vi "MAIN_SERVER.vi"() -> ()   [LabVIEW 2016]
uses:
  TypeDef/IN_Cluster.ctl
  TypeDef/OUT_CLUSTER.ctl
  <vilib>/DAQmx/read.llb/DAQmx Read (Analog 1D Wfm NChan NSamp).vi
  <vilib>/Analysis/baseanly.llb/Mean (DBL).vi
  <vilib>/DAQmx/miscellaneous.llb/DAQmx Fill In Error Info.vi
  <vilib>/Analysis/NI_AALBase.lvlib
  <vilib>/DAQmx/write.llb/DAQmx Write (Analog 1D DBL NChan 1Samp).vi
  <vilib>/DAQmx/read.llb/DAQmx Read (Analog 1D DBL NChan 1Samp).vi
  <vilib>/DAQmx/write.llb/DAQmx Write (Digital 1D Bool NChan 1Samp 1Line).vi
  <vilib>/DAQmx/read.llb/DAQmx Read (Digital 1D Bool NChan 1Samp 1Line).vi
panel:
  in  "Tab Control":enum32{"settings", "filtri AI ", "clusters"}(tab)
  in  "number of samples per channel":i32=500
  in  "rate":dbl=1000.0 format="%0.2f"
  out "Array nomi moduli":string[](array[string])
  in  "sample mode":i32(ring)=10123 items=["Finite Samples"=10178, "Continuous Samples"=10123, "Hardware Timed Single Point"=12522]
  in  "Impostazioni filtri digitali su AI":T1(array[cluster])=[{"filter?"=FALSE, "low cutoff freq: fl"=0.12500000000000006, "order"=2}, {"filter?"=FALSE, "low cutoff freq: fl"=0.12500000000000006, "order"=2}, {"filter?"=FALSE, "low cutoff freq: fl"=0.12500000000000006, "order"=2}, {"filter?"=FALSE, "low cutoff freq: fl"=0.12500000000000006, "order"=2}, {"filter?"=FALSE, "low cutoff freq: fl"=0.12500000000000006, "order"=2}, {"filter?"=FALSE, "low cutoff freq: fl"=0.12500000000000006, "order"=2}, {"filter?"=FALSE, "low cutoff freq: fl"=0.12500000000000006, "order"=2}, {"filter?"=FALSE, "low cutoff freq: fl"=0.12500000000000006, "order"=2}, {"filter?"=FALSE, "low cutoff freq: fl"=0.12500000000000006, "order"=2}, {"filter?"=FALSE, "low cutoff freq: fl"=0.12500000000000006, "order"=2}, {"filter?"=FALSE, "low cutoff freq: fl"=0.12500000000000006, "order"=2}, {"filter?"=FALSE, "low cutoff freq: fl"=0.12500000000000006, "order"=2}, {"filter?"=FALSE, "low cutoff freq: fl"=0.12500000000000006, "order"=2}, {"filter?"=FALSE, "low cutoff freq: fl"=0.12500000000000006, "order"=2}, {"filter?"=FALSE, "low cutoff freq: fl"=0.12500000000000006, "order"=2}, {"filter?"=FALSE, "low cutoff freq: fl"=0.12500000000000006, "order"=2}] {"low cutoff freq: fl" format="%0.4f"}
  out "AI Non filtrati":waveform(dbl)[](graph)
  out "AI filtrati":waveform(dbl)[](graph)
  out "Scritture":T2 {"AO" format="%f%0.2f"}
  in  "IN CLUSTER":T3 {"Stato uscite"."AO" format="%f%0.2f"; "AI2" format="%#_6f"; "TC" format="%#_4f"; "AI1" format="%#_6f"}
  in  "DO":bool[](array[boolean])
  in  "AO":dbl[](array[numeric]) format="%f%0.2f"
  in  "stop":bool
  # "AI"
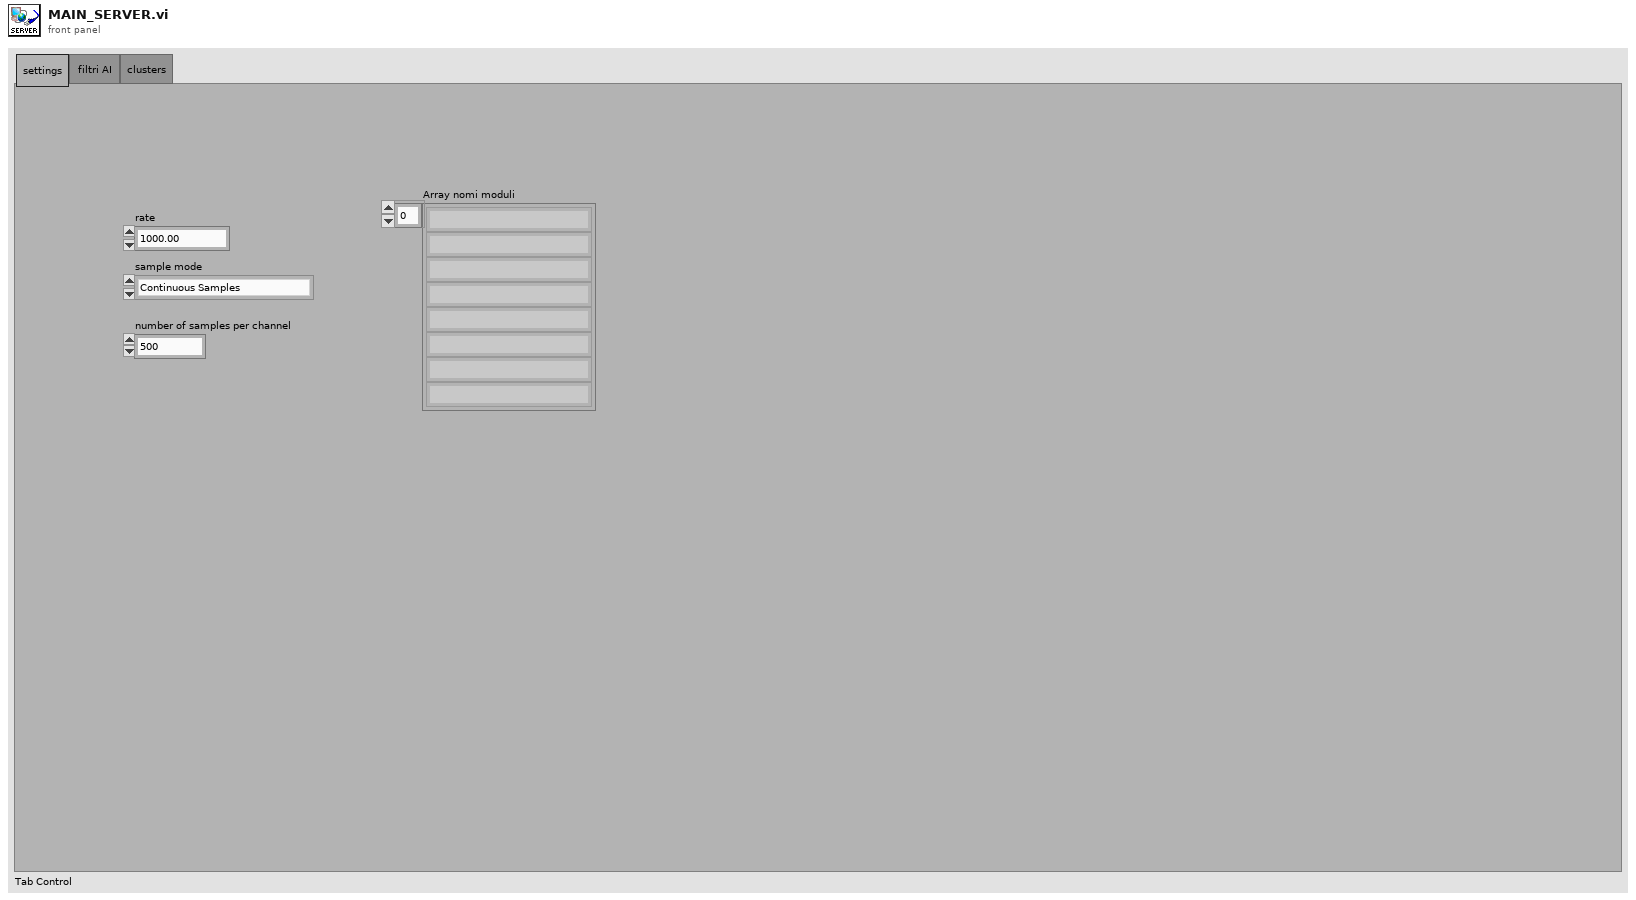
[diagram p1: front panel]
types:
  T1 = cluster{"filter?":bool, "low cutoff freq: fl":dbl, "order":i32}[]
  T2 = typedef "OUT_CLUSTER.ctl" = cluster{"DO ":bool[], "AO":dbl[], "Scelta banco PC1":dbl, "Scelta banco PC2":dbl, "Scelta ASP PC1":dbl, "Scelta ASP PC2":dbl, "Scelta MAND PC1":dbl, "Scelta MAND PC2":dbl, "Scelta Q PC1":dbl, "Scelta Q PC2":dbl}
  T3 = typedef "IN_Cluster.ctl" = cluster{"DI":bool[], "AI1":dbl[], "TC":dbl[], "AI2":dbl[], "Stato uscite":T2}
  T4 = cluster{"DI task":refnum<k21>, "DO task":refnum<k21>, "AI task":refnum<k21>, "AO task":refnum<k21>, "TC task":refnum<k21>}
  T5 = cluster{"Array of elements":cluster{"String":string, "variant":variant}[], "Single element":cluster{"String":string, "variant":variant}, "enque at\nopposite end (F)":bool, "no replications (F)":bool}
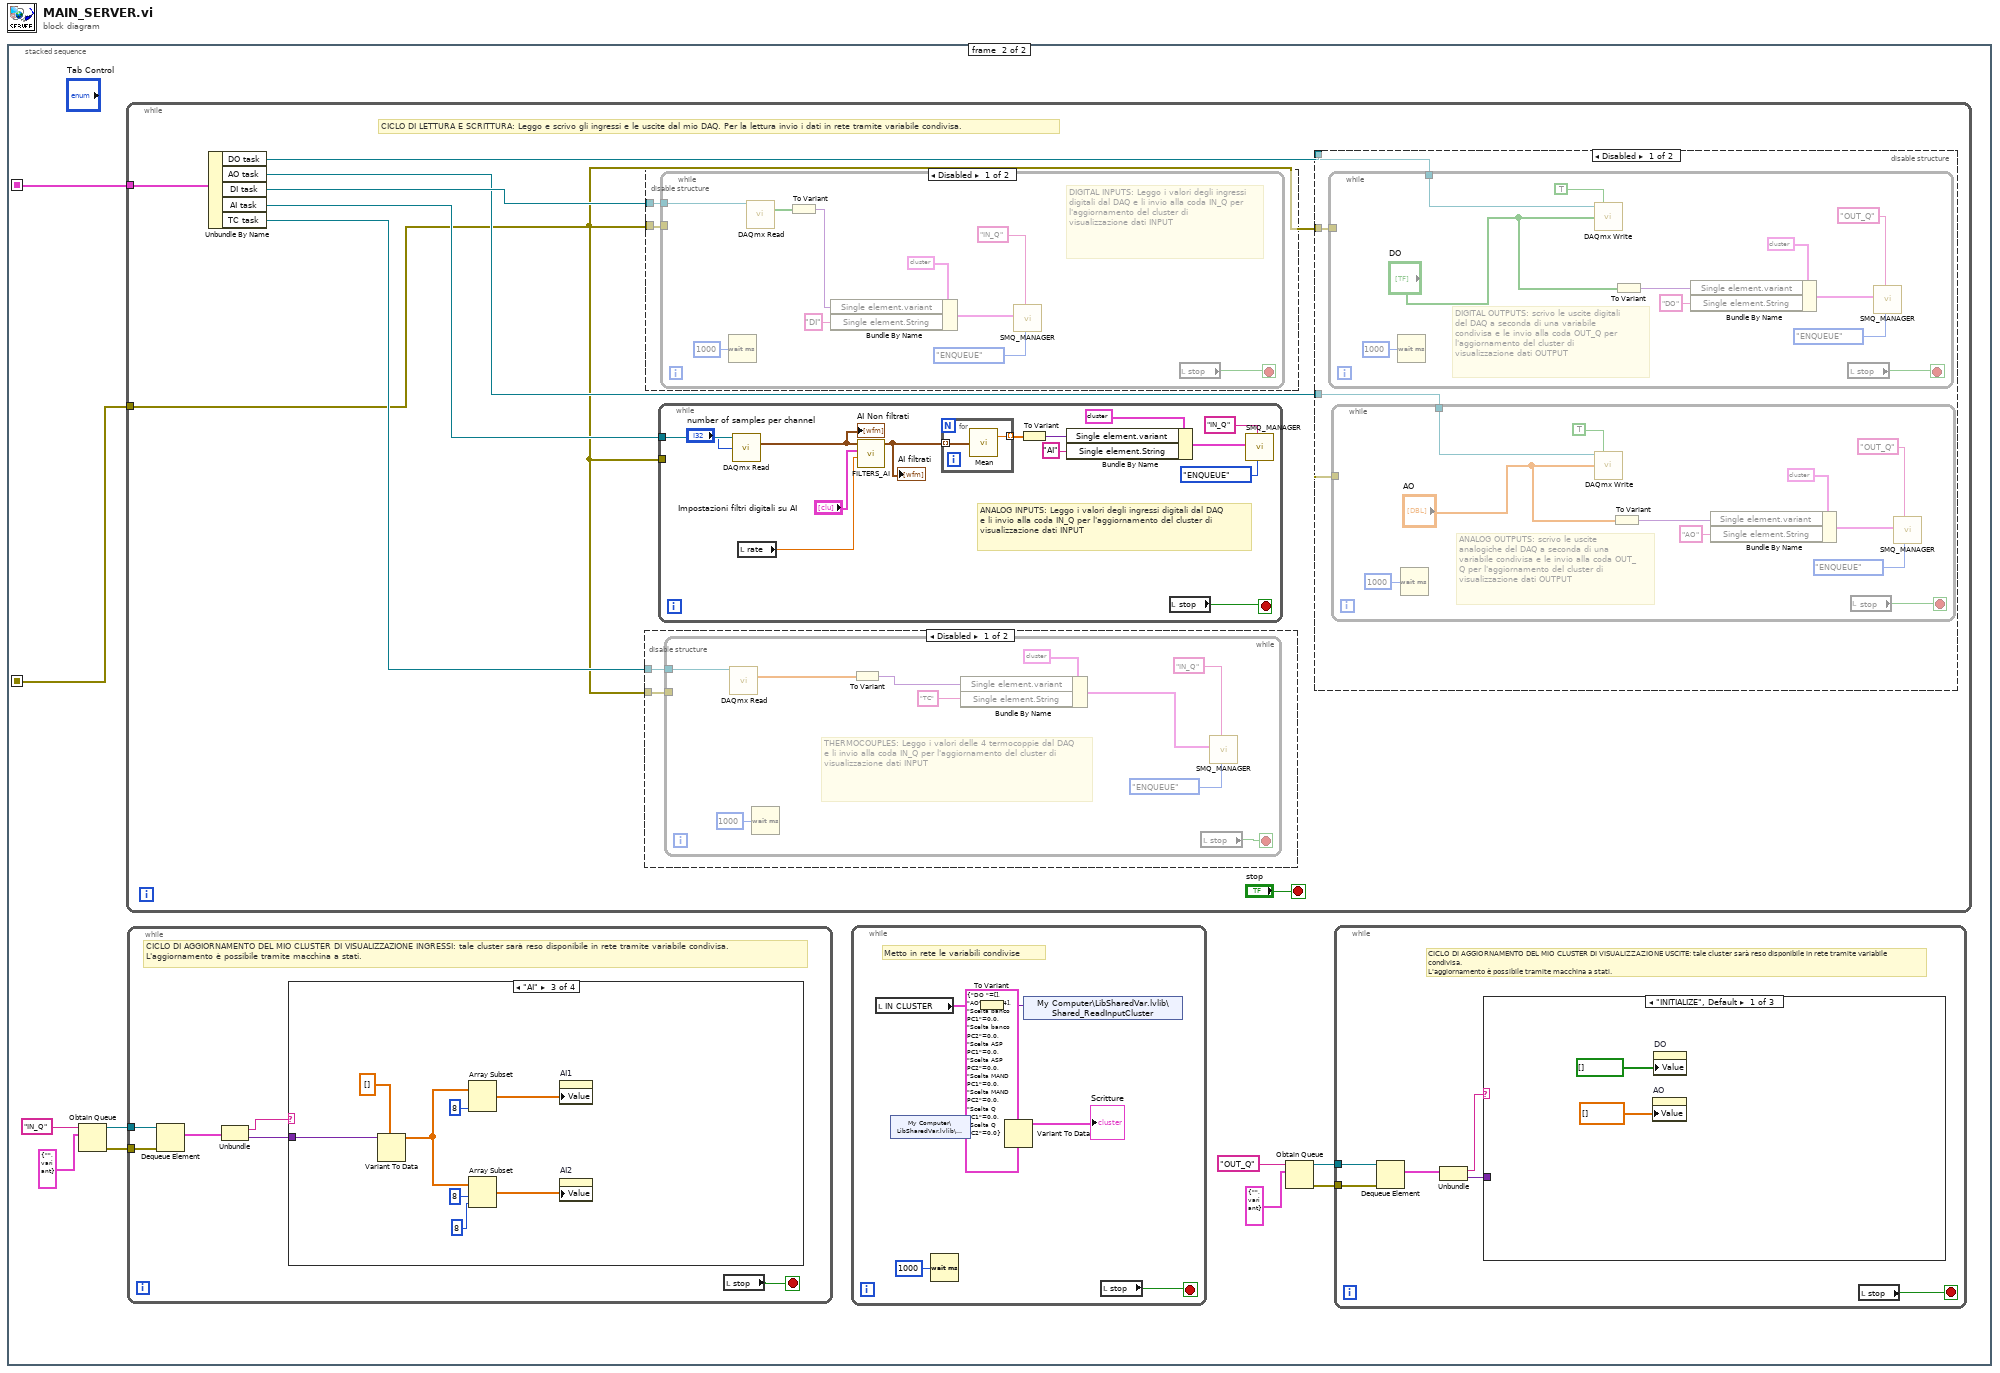
[diagram p0: block diagram]
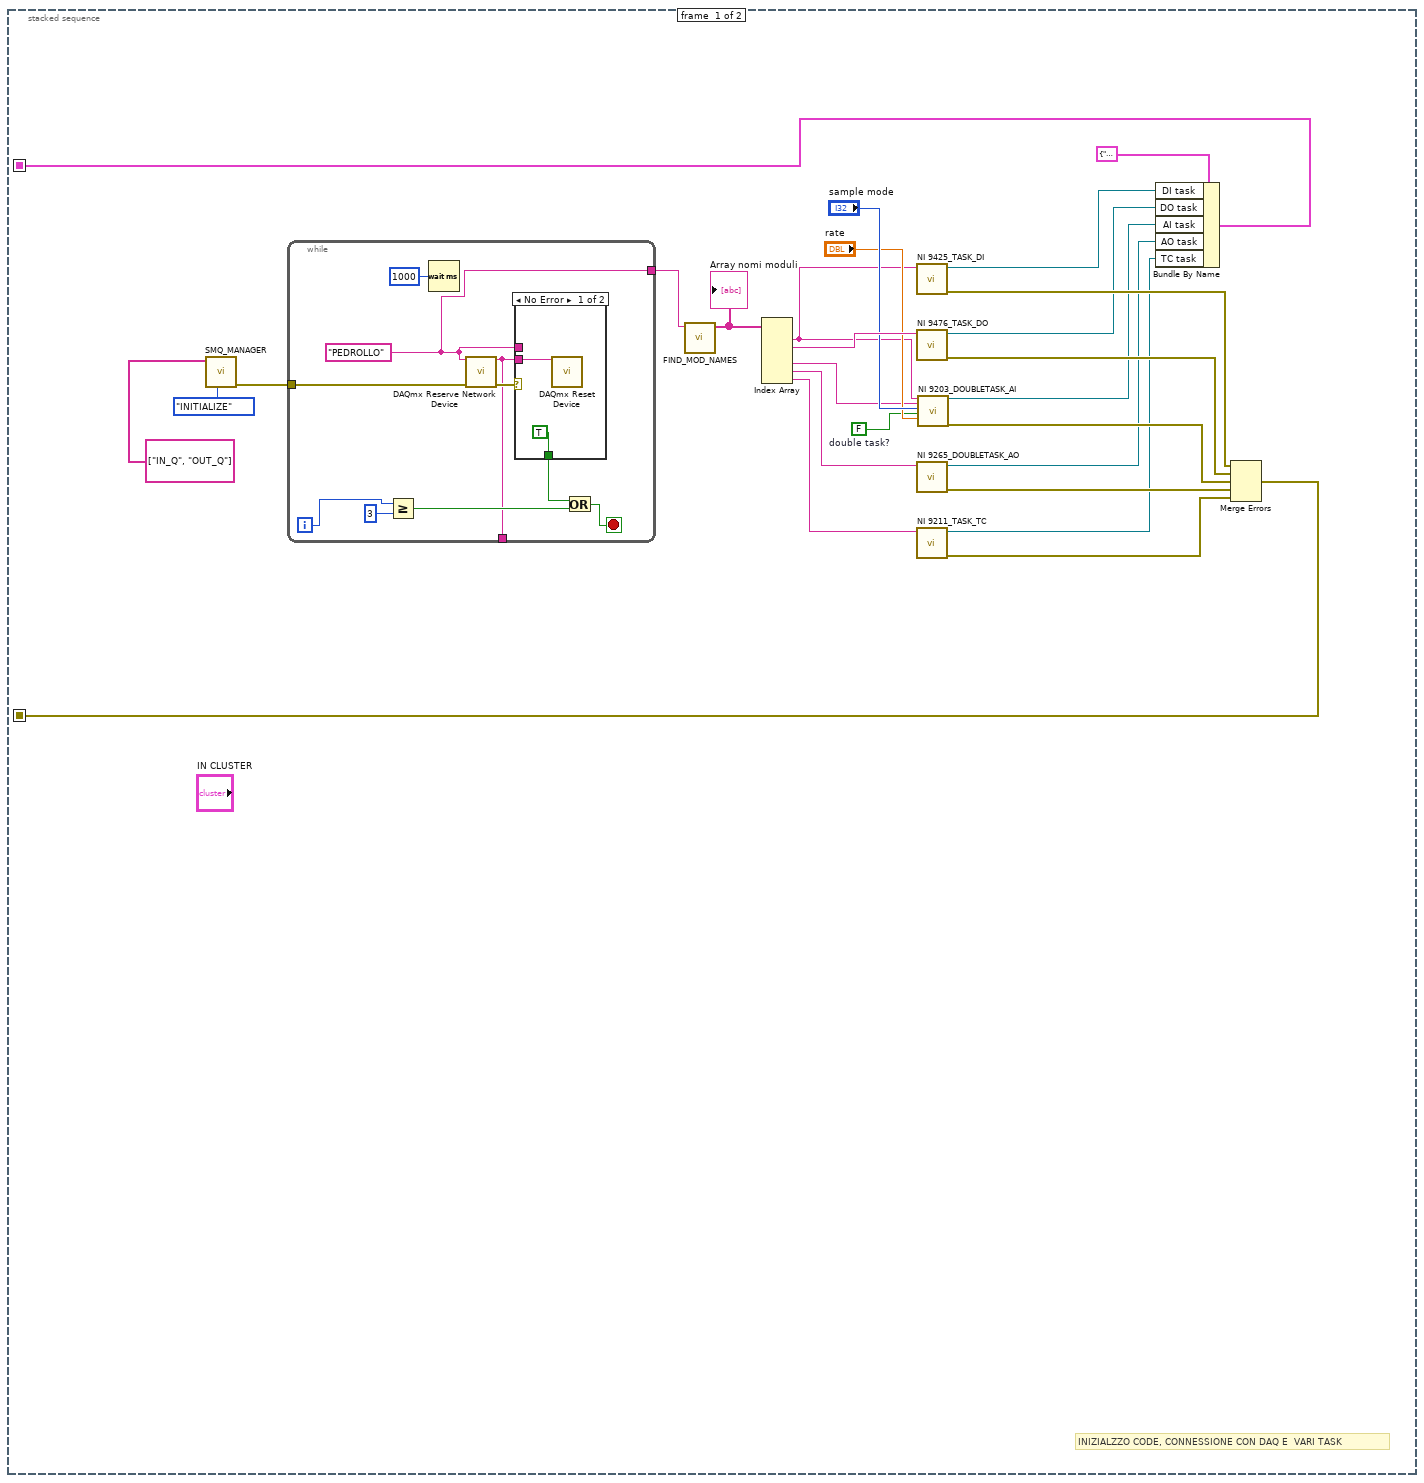
[diagram p2: hidden frame]
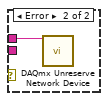
[diagram p3: hidden frame]
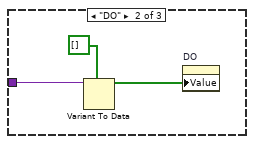
[diagram p4: hidden frame]
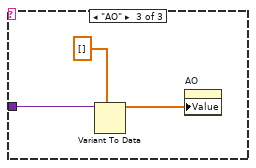
[diagram p5: hidden frame]
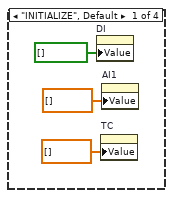
[diagram p6: hidden frame]
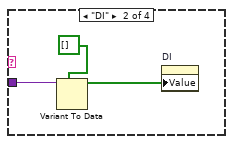
[diagram p7: hidden frame]
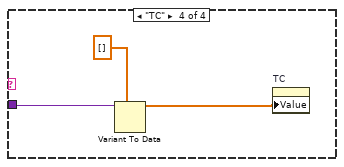
[diagram p8: hidden frame]
diagram:
  n1 = stacked-sequence {
    seq-local: [w16 _] -> [_ w49]
    seq-local: [w12 _] -> [_ w48]
    frame #0 {
      w2 = FALSE  # double task?
      # "INIZIALZZO CODE, CONNESSIONE CON DAQ E  VARI TASK"
      n2 = call <userlib>:"SMQ_MANAGER.vi"("Function"=enum16{"INITIALIZE", "ENQUEUE", "STOP ALL"}."INITIALIZE", "Queue array"=string[] ["IN_Q", "OUT_Q"]) -> ("error out"=w11:errorcluster)  [unwired: 9 in]
      n3 = while {
        tunnel: [w29] -> _
        tunnel: [w28] -> w17
        tunnel: w11 -> [w27]
        i -> [w34]
        stop <- w31 stop-if-true
        w28 = "PEDROLLO" ("RICERCA cDAQ")
        n4 = Greater Or Equal?(x=w34, y=3) -> (x >= y?=w32:bool)
        n5 = Wait (ms)(milliseconds to wait=u32 1000) -> ()  [unwired: 1 out]
        n6 = call <vilib>:"DAQmx Reserve Network Device.vi"("device in"=w28, "error in"=w27) -> ("device out"=w29:tag, "error out"=w36:errorcluster)  [unwired: 12 in]
        n7 = case shown="No Error" w36 {
          tunnel: w28 -> [_ w39]
          tunnel: [TRUE _] -> w35
          tunnel: w29 -> [w37 _]
          frame No Error {
            n8 = call <vilib>:"DAQmx Reset Device.vi"("device in"=w37) -> ()  [unwired: 14 in, 1 out]
          }
          frame Error {
            n9 = call <vilib>:"DAQmx Unreserve Network Device.vi"("device in"=w39) -> ()  [unwired: 13 in, 2 out]
          }
        }
        n10 = Or(x=w35, y=w32) -> (x .or. y?=w31:bool)
      }
      n11 = call "FIND_MOD_NAMES.vi"("RICERCA cDAQ"=w17) -> ("Array nomi moduli"=w23:string[])  [unwired: 7 in, 3 out]
      "Array nomi moduli" <- w23
      n12 = Index Array(array=w23) -> (element #1=w1:string, element #2=w24:string, element #4=w4:string, element #5=w6:string, element #6=w5:string)  [unwired: 6 in, 1 out]
      n13 = call "NI 9425_TASK_DI.vi"("MODULE NAME"=w1) -> ("error out"=w22:errorcluster, "task out"=w14:refnum<k21>)  [unwired: 9 in]
      n14 = call "NI 9476_TASK_DO.vi"("MODULE NAME"=w24) -> ("error out"=w21:errorcluster, "task out"=w13:refnum<k21>)  [unwired: 9 in]
      n15 = call "NI 9265_DOUBLETASK_AO.vi"("MODULE NAME"=w6) -> ("error out"=w19:errorcluster, "task out"=w9:refnum<k21>)  [unwired: 9 in]
      n16 = call "NI 9211_TASK_TC.vi"("MODULE NAME"=w5) -> ("error out"=w18:errorcluster, "task out"=w10:refnum<k21>)  [unwired: 9 in]
      n17 = call "NI 9203_DOUBLETASK_AI.vi"("MODULE NAME"=w1, "MODULE NAME 2"=w4, "sample mode"="sample mode", "double task?"=w2, "rate"="rate") -> ("task out"=w3:refnum<k21>, "error out"=w20:errorcluster)  [unwired: 13 in]
      n18 = Bundle By Name(cluster=T4 {"DI task"="", "DO task"="", "AI task"="", "AO task"="", "TC task"=""}, "DI task"=w14, "DO task"=w13, "AI task"=w3, "AO task"=w9, "TC task"=w10) -> (w12:T4)
      n19 = Merge Errors(w22, w21, w20, w19, w18) -> (w16:errorcluster)
    }
    frame #1 {
      n20 = Obtain Queue(name (unnamed)="IN_Q", element data type=cluster{"String":string, "variant":variant} {"String"="", "variant"=variant} ("element")) -> (queue out=w45:refnum<queue>, error out=w44:errorcluster)  [unwired: 3 in, 1 out]
      n21 = while {
        tunnel: w49 -> [w94]
        tunnel: w48 -> [w101]
        stop <- "stop" stop-if-true
        # "CICLO DI LETTURA E SCRITTURA: Leggo e scrivo gli ingressi e le uscite dal mio DAQ. Per la lettura invio i dati in rete tramite variabile condivisa."
        n22 = Unbundle By Name(w101) -> ("DO task"=w96:refnum<k21>, "AO task"=w95:refnum<k21>, "DI task"=w100:refnum<k21>, "AI task"=w97:refnum<k21>, "TC task"=w98:refnum<k21>)
        n23 = disable-structure shown="Disabled" {
          disable-tunnel: w98 -> [w115 _]
          disable-tunnel: w94 -> [w114 _]
          frame Disabled {
            n24 = while {
              tunnel: w114 -> [_]
              tunnel: w115 -> [w116]
              stop <- w117 stop-if-true
              # "THERMOCOUPLES: Leggo i valori delle 4 termocoppie dal DAQ e li invio alla coda IN_Q per l'aggiornamento del cluster di visualizzazione dati INPUT"
              n25 = call-poly <vilib>:"DAQmx Read.vi"("task/channels in"=w116) -> ("data"=w125:dbl[])  [unwired: 12 in, 2 out]
              n26 = Wait (ms)(milliseconds to wait=u32 1000) -> ()  [unwired: 1 out]
              n27 = To Variant(anything=w125) -> (Variant=w124:variant)
              n28 = Bundle By Name(cluster=T5 {"Array of elements"=[], "Single element"={"String"="", "variant"=variant}, "enque at\nopposite end (F)"=FALSE, "no replications (F)"=FALSE} ("Enqueue cluster"), "Single element.variant"=w124, "Single element.String"="TC") -> (w119:T5)
              n29 = local read "stop"() -> (w117:bool)
              n30 = call <userlib>:"SMQ_MANAGER.vi"("Function"=enum16{"INITIALIZE", "ENQUEUE", "STOP ALL"}."ENQUEUE", "Queue name"="IN_Q", "Enqueue cluster"=w119) -> ()  [unwired: 8 in, 1 out]
            }
          }
          frame Enabled {
          }
        }
        n31 = disable-structure shown="Disabled" {
          disable-tunnel: w100 -> [w103 _]
          disable-tunnel: w94 -> [w102 _]
          frame Disabled {
            n32 = while {
              tunnel: w102 -> [_]
              tunnel: w103 -> [w112]
              stop <- w104 stop-if-true
              # "DIGITAL INPUTS: Leggo i valori degli ingressi digitali dal DAQ e li invio alla coda IN_Q per l'aggiornamento del cluster di visualizzazione dati INPUT"
              n33 = Wait (ms)(milliseconds to wait=u32 1000) -> ()  [unwired: 1 out]
              n34 = call-poly <vilib>:"DAQmx Read.vi"("task/channels in"=w112) -> ("data"=w113:bool[])  [unwired: 12 in, 2 out]
              n35 = To Variant(anything=w113) -> (Variant=w110:variant)
              n36 = Bundle By Name(cluster=T5 {"Array of elements"=[], "Single element"={"String"="", "variant"=variant}, "enque at\nopposite end (F)"=FALSE, "no replications (F)"=FALSE} ("Enqueue cluster"), "Single element.variant"=w110, "Single element.String"="DI") -> (w109:T5)
              n37 = call <userlib>:"SMQ_MANAGER.vi"("Function"=enum16{"INITIALIZE", "ENQUEUE", "STOP ALL"}."ENQUEUE", "Queue name"="IN_Q", "Enqueue cluster"=w109) -> ()  [unwired: 8 in, 1 out]
              n38 = local read "stop"() -> (w104:bool)
            }
          }
          frame Enabled {
          }
        }
        n39 = while {
          tunnel: w94 -> [_]
          tunnel: w97 -> [w155]
          stop <- w156 stop-if-true
          # "ANALOG INPUTS: Leggo i valori degli ingressi digitali dal DAQ e li invio alla coda IN_Q per l'aggiornamento del cluster di visualizzazione dati INPUT"
          n40 = call-poly <vilib>:"DAQmx Read.vi"("task/channels in"=w155, "number of samples per channel"="number of samples per channel") -> ("data"=w153:waveform(dbl)[])  [unwired: 11 in, 2 out]
          "AI Non filtrati" <- w153
          n41 = local read "rate"() -> (w151:dbl)
          n42 = call "FILTERS_AI.vi"("sampling freq: fs"=w151, "Array"="Impostazioni filtri digitali su AI", "data in"=w153) -> ("filtered"=w152:waveform(dbl)[])  [unwired: 8 in]
          "AI filtrati" <- w152
          n43 = for {
            tunnel: [w166] -> w158 mode=indexing
            tunnel: w152 -> [w165] mode=indexing
            n44 = call-poly <vilib>:"Mean.vi"("X"=w165) -> ("mean"=w166:dbl)  [unwired: 1 out]
          }
          n45 = To Variant(anything=w158) -> (Variant=w157:variant)
          n46 = Bundle By Name(cluster=T5 {"Array of elements"=[], "Single element"={"String"="", "variant"=variant}, "enque at\nopposite end (F)"=FALSE, "no replications (F)"=FALSE} ("Enqueue cluster"), "Single element.variant"=w157, "Single element.String"="AI") -> (w163:T5)
          n47 = local read "stop"() -> (w156:bool)
          n48 = call <userlib>:"SMQ_MANAGER.vi"("Function"=enum16{"INITIALIZE", "ENQUEUE", "STOP ALL"}."ENQUEUE", "Queue name"="IN_Q", "Enqueue cluster"=w163) -> ()  [unwired: 8 in, 1 out]
        }
        n49 = disable-structure shown="Disabled" {
          disable-tunnel: w96 -> [w128 _]
          disable-tunnel: w95 -> [w127 _]
          disable-tunnel: w94 -> [w126 _]
          frame Disabled {
            n50 = while {
              tunnel: w128 -> [w148]
              tunnel: w126 -> [_]
              stop <- w149 stop-if-true
              # "DIGITAL OUTPUTS: scrivo le uscite digitali del DAQ a seconda di una variabile condivisa e le invio alla coda OUT_Q per l'aggiornamento del cluster di visualizzazione dati OUTPUT"
              n51 = Wait (ms)(milliseconds to wait=u32 1000) -> ()  [unwired: 1 out]
              n52 = call-poly <vilib>:"DAQmx Write.vi"("task/channels in"=w148, "auto start"=TRUE, "data"="DO") -> ()  [unwired: 10 in, 3 out]
              n53 = To Variant(anything="DO") -> (Variant=w143:variant)
              n54 = Bundle By Name(cluster=T5 {"Array of elements"=[], "Single element"={"String"="", "variant"=variant}, "enque at\nopposite end (F)"=FALSE, "no replications (F)"=FALSE} ("Enqueue cluster"), "Single element.variant"=w143, "Single element.String"="DO") -> (w144:T5)
              n55 = local read "stop"() -> (w149:bool)
              n56 = call <userlib>:"SMQ_MANAGER.vi"("Function"=enum16{"INITIALIZE", "ENQUEUE", "STOP ALL"}."ENQUEUE", "Queue name"="OUT_Q", "Enqueue cluster"=w144) -> ()  [unwired: 8 in, 1 out]
            }
            n57 = while {
              tunnel: w127 -> [w137]
              tunnel: w126 -> [_]
              stop <- w138 stop-if-true
              # "ANALOG OUTPUTS: scrivo le uscite analogiche del DAQ a seconda di una variabile condivisa e le invio alla coda OUT_Q per l'aggiornamento del cluster di visualizzazione dati OUTPUT"
              n58 = Wait (ms)(milliseconds to wait=u32 1000) -> ()  [unwired: 1 out]
              n59 = call-poly <vilib>:"DAQmx Write.vi"("task/channels in"=w137, "auto start"=TRUE, "data"="AO") -> ()  [unwired: 10 in, 3 out]
              n60 = To Variant(anything="AO") -> (Variant=w130:variant)
              n61 = Bundle By Name(cluster=T5 {"Array of elements"=[], "Single element"={"String"="", "variant"=variant}, "enque at\nopposite end (F)"=FALSE, "no replications (F)"=FALSE} ("Enqueue cluster"), "Single element.variant"=w130, "Single element.String"="AO") -> (w133:T5)
              n62 = local read "stop"() -> (w138:bool)
              n63 = call <userlib>:"SMQ_MANAGER.vi"("Function"=enum16{"INITIALIZE", "ENQUEUE", "STOP ALL"}."ENQUEUE", "Queue name"="OUT_Q", "Enqueue cluster"=w133) -> ()  [unwired: 8 in, 1 out]
            }
          }
          frame Enabled {
          }
        }
      }
      n64 = while {
        tunnel: w45 -> [w75]
        tunnel: w44 -> [w74]
        stop <- w76 stop-if-true
        # "CICLO DI AGGIORNAMENTO DEL MIO CLUSTER DI VISUALIZZAZIONE INGRESSI: tale cluster sarà reso disponibile in rete tramite variabile condivisa.\nL'aggiornamento è possibile tramite macchina a stati."
        n65 = Dequeue Element(queue=w75, error in (no error)=w74) -> (element=w73:cluster{"String":string, "variant":variant})  [unwired: 1 in, 3 out]
        n66 = Unbundle(w73) -> ("String"=w72:string, "variant"=w71:variant)
        n67 = case shown="\"AI\"" w72 {
          tunnel: w71 -> [_ w82 w90 w92]
          frame "INITIALIZE", Default {
            n68 = property on="DI" class="Arr (strict)"("Value"=bool[] []) -> ()  [unwired: 2 in, 2 out]
            n69 = property on="TC" class="Arr (strict)"("Value"=dbl[] []) -> ()  [unwired: 2 in, 2 out]
            n70 = property on="AI1" class="Arr (strict)"("Value"=dbl[] []) -> ()  [unwired: 2 in, 2 out]
          }
          frame "DI" {
            n71 = Variant To Data(type=bool[] [], Variant=w82) -> (data=w80:bool[])  [unwired: 1 in, 1 out]
            n72 = property on="DI" class="Arr (strict)"("Value"=w80) -> ()  [unwired: 2 in, 2 out]
          }
          frame "AI" {
            n73 = Variant To Data(type=dbl[] [], Variant=w90) -> (data=w88:dbl[])  [unwired: 1 in, 1 out]
            n74 = Array Subset(array=w88, length=8) -> (w87:dbl[])  [unwired: 1 in]
            n75 = Array Subset(array=w88, index=8, length=8) -> (w86:dbl[])
            n76 = property on="AI1" class="Arr (strict)"("Value"=w87) -> ()  [unwired: 2 in, 2 out]
            n77 = property on="AI2" class="Arr (strict)"("Value"=w86) -> ()  [unwired: 2 in, 2 out]
          }
          frame "TC" {
            n78 = Variant To Data(type=dbl[] [], Variant=w92) -> (data=w91:dbl[])  [unwired: 1 in, 1 out]
            n79 = property on="TC" class="Arr (strict)"("Value"=w91) -> ()  [unwired: 2 in, 2 out]
          }
        }
        n80 = local read "stop"() -> (w76:bool)
      }
      n81 = while {
        stop <- w67 stop-if-true
        # "Metto in rete le variabili condivise"
        n82 = local read "IN CLUSTER"() -> (w69:T3)
        n83 = shared-variable "My Computer\\LibSharedVar.lvlib\\Scritture"() -> (w66:variant)  [unwired: 1 in, 1 out]
        n84 = Wait (ms)(milliseconds to wait=u32 1000) -> ()  [unwired: 1 out]
        n85 = To Variant(anything=w69) -> (Variant=w70:variant)
        n86 = Variant To Data(type=T2 {"DO "=[], "AO"=[0.004], "Scelta banco PC1"=0.0, "Scelta banco PC2"=0.0, "Scelta ASP PC1"=0.0, "Scelta ASP PC2"=0.0, "Scelta MAND PC1"=0.0, "Scelta MAND PC2"=0.0, "Scelta Q PC1"=0.0, "Scelta Q PC2"=0.0} ("Scritture"), Variant=w66) -> (data=→"Scritture":T2)  [unwired: 1 in, 1 out]
        n87 = shared-variable "My Computer\\LibSharedVar.lvlib\\Shared_ReadInputCluster"(w70) -> ()  [unwired: 1 in, 1 out]
        n88 = local read "stop"() -> (w67:bool)
      }
      n89 = Obtain Queue(name (unnamed)="OUT_Q", element data type=cluster{"String":string, "variant":variant} {"String"="", "variant"=variant} ("element")) -> (queue out=w41:refnum<queue>, error out=w40:errorcluster)  [unwired: 3 in, 1 out]
      n90 = while {
        tunnel: w41 -> [w54]
        tunnel: w40 -> [w53]
        stop <- w55 stop-if-true
        # "CICLO DI AGGIORNAMENTO DEL MIO CLUSTER DI VISUALIZZAZIONE USCITE: tale cluster sarà reso disponibile in rete tramite variabile condivisa.\nL'aggiornamento è possibile tramite macchina a stati."
        n91 = Dequeue Element(queue=w54, error in (no error)=w53) -> (element=w52:cluster{"String":string, "variant":variant})  [unwired: 1 in, 3 out]
        n92 = Unbundle(w52) -> ("String"=w51:string, "variant"=w50:variant)
        n93 = case shown="\"INITIALIZE\", Default" w51 {
          tunnel: w50 -> [_ w59 w62]
          frame "INITIALIZE", Default {
            n94 = property on="AO" class="Arr (strict)"("Value"=dbl[] []) -> ()  [unwired: 2 in, 2 out]
            n95 = property on="DO" class="Arr (strict)"("Value"=bool[] []) -> ()  [unwired: 2 in, 2 out]
          }
          frame "DO" {
            n96 = Variant To Data(type=bool[] [], Variant=w59) -> (data=w58:bool[])  [unwired: 1 in, 1 out]
            n97 = property on="DO" class="Arr (strict)"("Value"=w58) -> ()  [unwired: 2 in, 2 out]
          }
          frame "AO" {
            n98 = Variant To Data(type=dbl[] [], Variant=w62) -> (data=w61:dbl[])  [unwired: 1 in, 1 out]
            n99 = property on="AO" class="Arr (strict)"("Value"=w61) -> ()  [unwired: 2 in, 2 out]
          }
        }
        n100 = local read "stop"() -> (w55:bool)
      }
    }
  }
